vi "gjson_ScanItem.vi"(6 "Offset In":i32, 7 "FlattenedData":string, 8 "error in":errorcluster, 10 "Disable Parse?":bool, 11 "variant":variant) -> (0 "error out":errorcluster, 2 "Enum?":bool, 3 "DataString":string, 4 "Offset Out":i32)   [LabVIEW 2015, in "Json2Labv.lvlib"]
uses:
  Json2Labv.lvlib
  <vilib>/Utility/VariantDataType/VariantType.lvlib
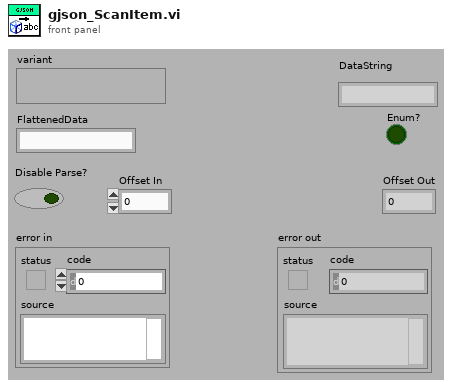
[diagram p1: front panel]
types:
  T1 = typedef "VariantType.lvlib/Type.ctl" = enum8{"Invalid Type", "Void", "I8", "I16", "I32", "I64", "U8", "U16", "U32", "U64", "Single Float", "Double Float", "Extended Float", "Single Complex", "Double Complex", "Extended Complex", "Enum U8", "Enum U16", "Enum U32", "Enum U64", "Single Float With Unit", "Double Float With Unit", "Extended Float With Unit", "Single Complex with Unit", "Double Complex with Unit", "Extended Complex with Unit", "Boolean", "String", "Path", "Picture", "Tag", "Array", "Cluster", "Variant", "LV Variant", "Waveform", "Timestamp", "Digital Waveform", "Digital Data", "ExpressData", "Refnum", "External Data", "VI", "Poly VI", "LabVIEW Class Instance", "Fixed Point"}
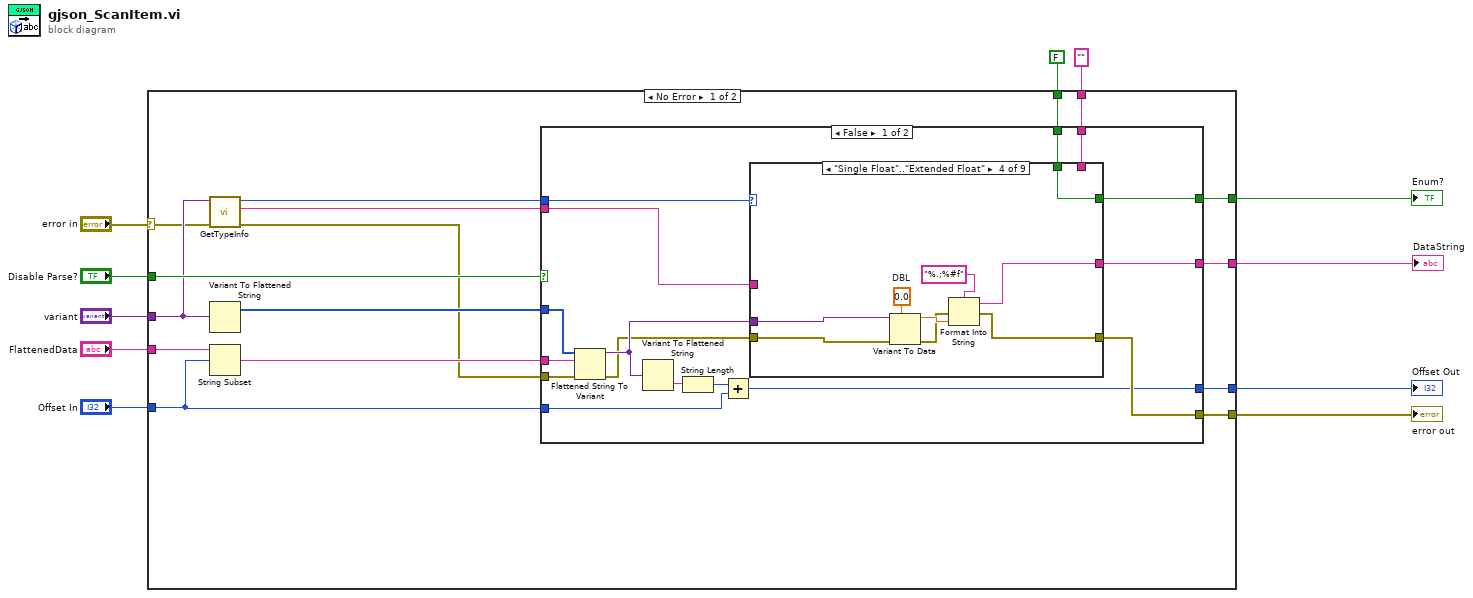
[diagram p0: block diagram]
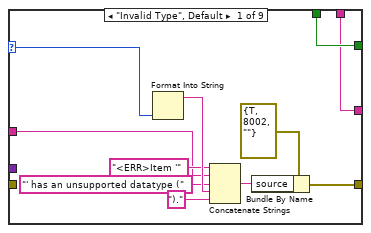
[diagram p2: hidden frame]
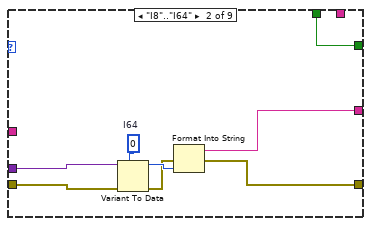
[diagram p3: hidden frame]
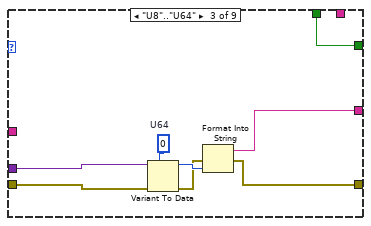
[diagram p4: hidden frame]
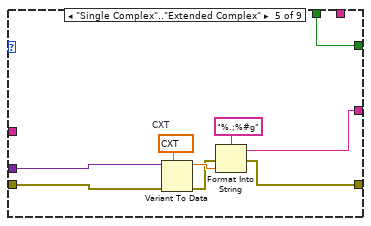
[diagram p5: hidden frame]
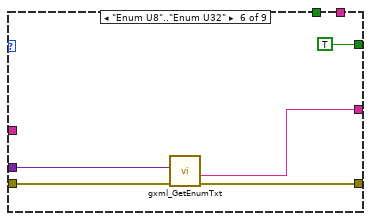
[diagram p6: hidden frame]
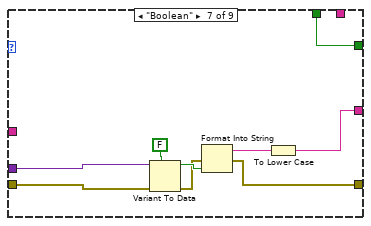
[diagram p7: hidden frame]
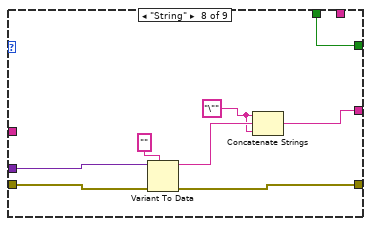
[diagram p8: hidden frame]
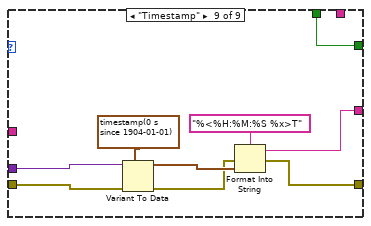
[diagram p9: hidden frame]
diagram:
  n1 = case shown="No Error" "error in" {
    selector: "error in" -> [w17 w126]
    tunnel: [w27 w126] -> w11
    tunnel: "Offset In" -> [w26 w127]
    tunnel: [w25 w127] -> w9
    tunnel: [w24 w125] -> w8
    tunnel: [w23 w124] -> w1
    tunnel: "Disable Parse?" -> [w21 _]
    tunnel: "FlattenedData" -> [w19 _]
    tunnel: "variant" -> [w18 _]
    tunnel: "" -> [w16 w124]
    tunnel: FALSE -> [w15 w125]
    frame No Error {
      n2 = call <vilib>:"GetTypeInfo.vi"("error in (no error)"=w17, "Variant"=w18) -> ("error out"=w12:errorcluster, "Name"=w13:string, "Type Enum"=w14:T1)  [unwired: 5 in, 2 out]
      n3 = Variant To Flattened String(Variant=w18) -> (1:w20:i16[])  [unwired: 1 out]
      n4 = String Subset(string=w19, offset (0)=w26) -> (substring=w22:string)  [unwired: 1 in]
      n5 = case shown="False" w21 {
        tunnel: w12 -> [w43 w122]
        tunnel: [w42 w122] -> w27
        tunnel: w26 -> [w41 w123]
        tunnel: [w40 w123] -> w25
        tunnel: w20 -> [w39 _]
        tunnel: [w38 w121] -> w24
        tunnel: [w28 w120] -> w23
        tunnel: w22 -> [w33 _]
        tunnel: w14 -> [w32 _]
        tunnel: w16 -> [w31 w120]
        tunnel: w15 -> [w30 w121]
        tunnel: w13 -> [w29 _]
        frame False {
          n6 = Flattened String To Variant(4:w43, 6:w33, 7:w39) -> (0:w34:errorcluster, 3:w35:variant)
          n7 = Variant To Flattened String(Variant=w35) -> (data string=w37:string)  [unwired: 1 out]
          n8 = String Length(string=w37) -> (length=w36:i32)
          n9 = Add(x=w36, y=w41) -> (x+y=w40:i32)
          n10 = case shown="\"Single Float\"..\"Extended Float\"" w32 {
            selector: w32 -> [w53 _ _ _ _ _ _ _ _]
            tunnel: w35 -> [_ w62 w69 w78 w86 w92 w102 w110 w115]
            tunnel: w34 -> [_ w55 w63 w77 w85 w89 w101 w106 w114]
            tunnel: [w54 w58 w66 w74 w83 w91 w97 w108 w113] -> w42
            tunnel: [w48 w57 w65 w73 w80 w90 w94 w105 w111] -> w28
            tunnel: [w49 w56 w64 w72 w81 TRUE w96 w107 w119] -> w38
            tunnel: w30 -> [w49 w56 w64 w72 w81 _ w96 w107 w119]
            tunnel: w31 -> [w48 _ _ _ _ _ _ _ _]
            tunnel: w29 -> [w46 _ _ _ _ _ _ _ _]
            frame "Invalid Type", Default {
              n11 = Format Into String(w53) -> (resulting string=w50:string)  [unwired: 3 in, 1 out]
              n12 = Concatenate Strings("<ERR>Item '" ("Format String"), w46, "' has an unsupported datatype (" ("Format String"), w50, ")." ("string")) -> (w51:string)
              n13 = Bundle By Name(cluster=errorcluster {"status"=TRUE, "code"=8002, "source"=""} ("error in"), "source"=w51) -> (w54:errorcluster)
            }
            frame "I8".."I64" {
              w61 = i64 0  # I64
              n14 = Variant To Data(error in=w55, type=w61, Variant=w62) -> (data=w60:i64, error out=w59:errorcluster)
              n15 = Format Into String(error in=w59, w60) -> (resulting string=w57:string, error out=w58:errorcluster)  [unwired: 2 in]
            }
            frame "U8".."U64" {
              w70 = u64 0  # U64
              n16 = Variant To Data(error in=w63, type=w70, Variant=w69) -> (data=w68:u64, error out=w67:errorcluster)
              n17 = Format Into String(error in=w67, w68) -> (resulting string=w65:string, error out=w66:errorcluster)  [unwired: 2 in]
            }
            frame "Single Float".."Extended Float" {
              w79 = 0.0  # DBL
              n18 = Variant To Data(error in=w77, type=w79, Variant=w78) -> (data=w76:dbl, error out=w75:errorcluster)
              n19 = Format Into String(format string="%.;%#f", error in=w75, w76) -> (resulting string=w73:string, error out=w74:errorcluster)  [unwired: 1 in]
            }
            frame "Single Complex".."Extended Complex" {
              w88 = cxt 0.0+0.0i  # CXT
              n20 = Variant To Data(error in=w85, type=w88, Variant=w86) -> (data=w87:cxt, error out=w84:errorcluster)
              n21 = Format Into String(format string="%.;%#g", error in=w84, w87) -> (resulting string=w80:string, error out=w83:errorcluster)  [unwired: 1 in]
            }
            frame "Enum U8".."Enum U32" {
              n22 = call "gxml_GetEnumTxt.vi"("error in"=w89, "Enum"=w92) -> ("error out"=w91:errorcluster, "String Value"=w90:string)  [unwired: 7 in, 1 out]
            }
            frame "Boolean" {
              n23 = Variant To Data(error in=w101, type=FALSE, Variant=w102) -> (data=w99:bool, error out=w98:errorcluster)
              n24 = Format Into String(error in=w98, w99) -> (resulting string=w95:string, error out=w97:errorcluster)  [unwired: 2 in]
              n25 = To Lower Case(string=w95) -> (all lower case string=w94:string)
            }
            frame "String" {
              w103 = "\"" ("string")
              n26 = Variant To Data(error in=w106, type="", Variant=w110) -> (data=w104:string, error out=w108:errorcluster)
              n27 = Concatenate Strings(w103, w104, w103) -> (w105:string)
            }
            frame "Timestamp" {
              n28 = Variant To Data(error in=w114, type=timestamp(0 s since 1904-01-01) ("time stamp"), Variant=w115) -> (data=w117:timestamp, error out=w116:errorcluster)
              n29 = Format Into String(format string="%<%H:%M:%S %x>T", error in=w116, w117) -> (resulting string=w111:string, error out=w113:errorcluster)  [unwired: 1 in]
            }
          }
        }
        frame True {
        }
      }
    }
    frame Error {
    }
  }
  "error out" <- w11
  "Offset Out" <- w9
  "Enum?" <- w8
  "DataString" <- w1
